vi "Config From YAML.vi"(8 "error in (no error)":errorcluster, 10 "YAML":string) -> (0 "error out":errorcluster, 2 "Config":refnum<class "Config Manager.lvclass">)   [LabVIEW 2020, in "CDM-Config.lvlib" / "Config-YAML.lvclass"]
uses:
  Config-YAML.lvclass
  Config-YAML.lvclass/Config-YAML.ctl
  Parser State.ctl
  Config Manager/Config Manager.lvclass
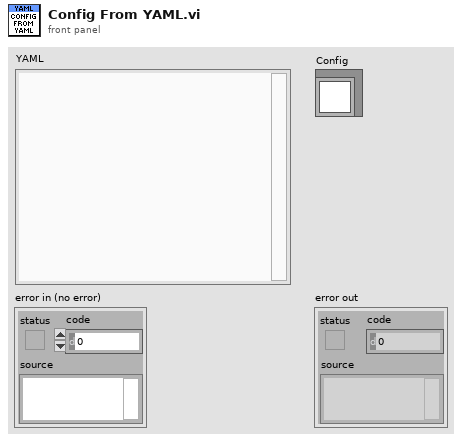
[diagram p1: front panel]
types:
  T1 = typedef "CDM-Config.lvlib/Config-YAML.lvclass/Parser State.ctl" = cluster{"YAML":string, "Indentation":i32[], "Hierarchy":string[], "Sequence Order":i32, "Offset":i32}
  T2 = typedef "CDM-Config.lvlib/Config Element.ctl" = cluster{"Hierarchy":string[], "Value":variant, "Meta Data":T3[], "Value Type":T4, "Child Order":i32}
  T3 = typedef "CDM-Config.lvlib/Meta Data.ctl" = cluster{"Name":string, "Value":string}
  T4 = typedef "CDM-Config.lvlib/Value Type.ctl" = enum16{"String", "Number", "Bool", "Object", "Array"}
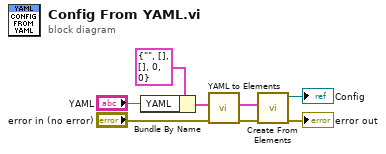
[diagram p0: block diagram]
diagram:
  n1 = Bundle By Name(cluster=T1 {"YAML"="", "Indentation"=[], "Hierarchy"=[], "Sequence Order"=0, "Offset"=0} ("Parser State"), "YAML"="YAML") -> (w1:T1)
  n2 = call "YAML to Elements.vi"("error in (no error)"="error in (no error)", "Parser State"=w1) -> ("error out"=w7:errorcluster, "Elements"=w6:T2[])  [unwired: 8 in]
  n3 = call "Create From Elements.vi"("error in (no error)"=w7, "Elements"=w6) -> ("error out"=→"error out":errorcluster, "Config Manager out"=→"Config":refnum<class "Config Manager.lvclass">)  [unwired: 8 in]
